vi "Get_DI.vi"(0 "reference in":refnum<class "Sig_DI_Simple.lvclass">) -> (6 "DI":bool)   [LabVIEW 2019, in "Sig_DI_Simple.lvclass"]
uses:
  Sig_DI_Simple.lvclass
  Sig_DI_Simple.lvclass/Sig_DI_Simple.ctl
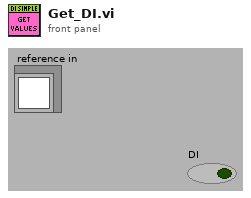
[diagram p1: front panel]
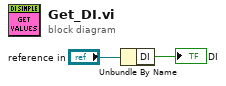
[diagram p0: block diagram]
diagram:
  n1 = Unbundle By Name("reference in") -> ("DI"=→"DI":bool)
